vi "test_Add Response_Variable Names Error.vi"(8 "error in (no error)":errorcluster, 11 "TestCase in":refnum<class "Instrument Addon Scripting API Messages Unit Tests.lvclass">) -> (0 "error out":errorcluster, 3 "TestCase out":refnum<class "Instrument Addon Scripting API Messages Unit Tests.lvclass">)   [LabVIEW 2018, in "Instrument Addon Scripting API Messages Unit Tests.lvclass"]
uses:
  Instrument Addon Scripting API Messages Unit Tests.lvclass
  APIs/Scripting API/TypeDefs/Wait Response Settings.ctl
  APIs/Scripting API/TypeDefs/Linked Channel.ctl
  <vilib>/NI Veristand/Custom Device API/Custom Device Item Ref.ctl
  Addon/Addon Shared/SubVIs/Constants.vi
  <vilib>/NI/NI VeriStand Advanced SysDef API/_SubVIs/SysDef.Search.GUID.vi
  APIs/Scripting API/Messages/Add Response - Wait (sec).vi
  <vilib>/addons/_JKI Toolkits/VI Tester/TestCase.llb/TestCase.lvclass
  Instrument Addon Scripting API Test Assets/Instrument Addon Scripting API Test Assets.lvclass
  APIs/Scripting API/Instrument Addon Scripting API.lvlib
  <vilib>/NI Veristand/Custom Device API/Custom Device API.lvlib
  <vilib>/NI/NI VeriStand Advanced SysDef API/SysDef API/Advanced System Definition.lvlib
  Addon/Addon Shared/Instrument Addon Shared.lvlib
  C:/Program Files (x86)/National Instruments/LabVIEW 2018/vi.lib/addons/_JKI Toolkits/VI Tester/TestCase.llb/TestCase.lvclass
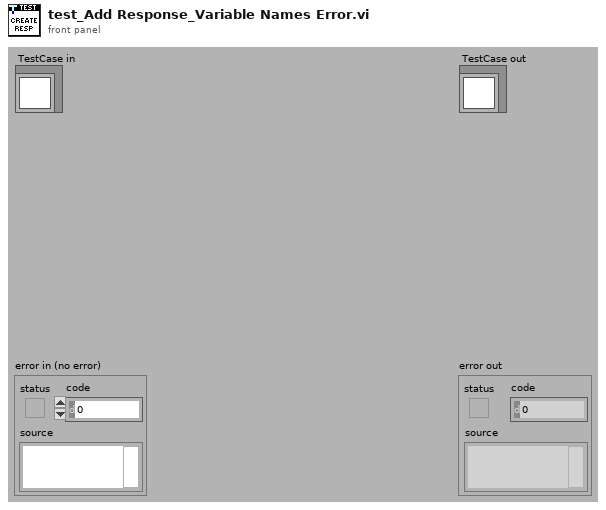
[diagram p1: front panel]
types:
  T1 = typedef "Instrument Addon Scripting API.lvlib/Wait Response Settings.ctl" = cluster{"Response Format":string, "Linked Channels":T2[], "Wait value (sec)":dbl, "Use Wait Channel":bool, "Channel Refnum":T3}
  T2 = typedef "Instrument Addon Scripting API.lvlib/Linked Channel.ctl" = cluster{"Variable Name":string, "Channel Refnum":T3}
  T3 = typedef "Custom Device API.lvlib/Custom Device Item Ref.ctl" = u64
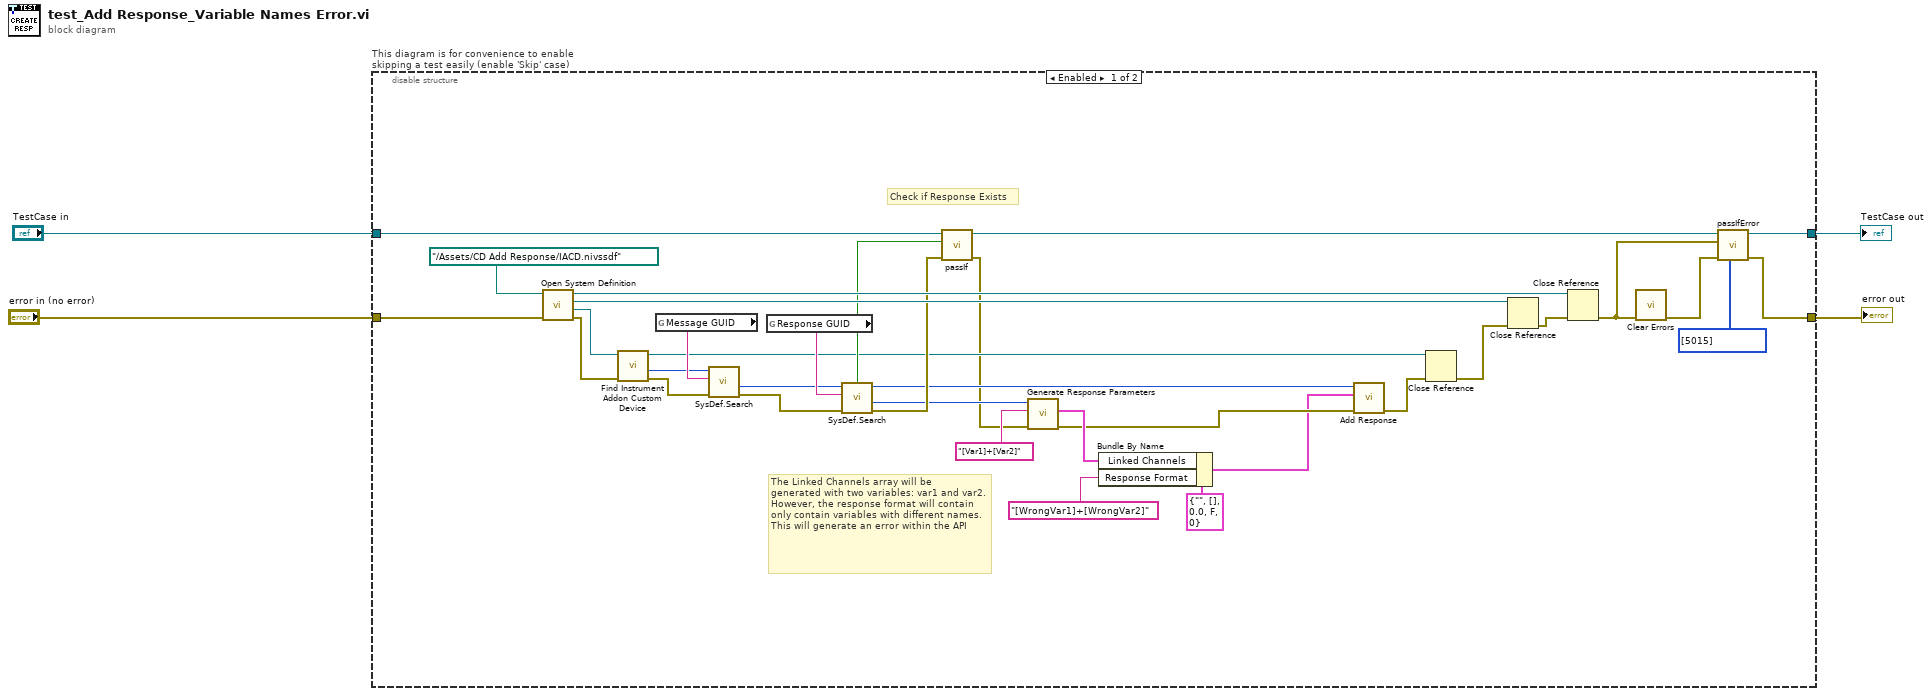
[diagram p0: block diagram]
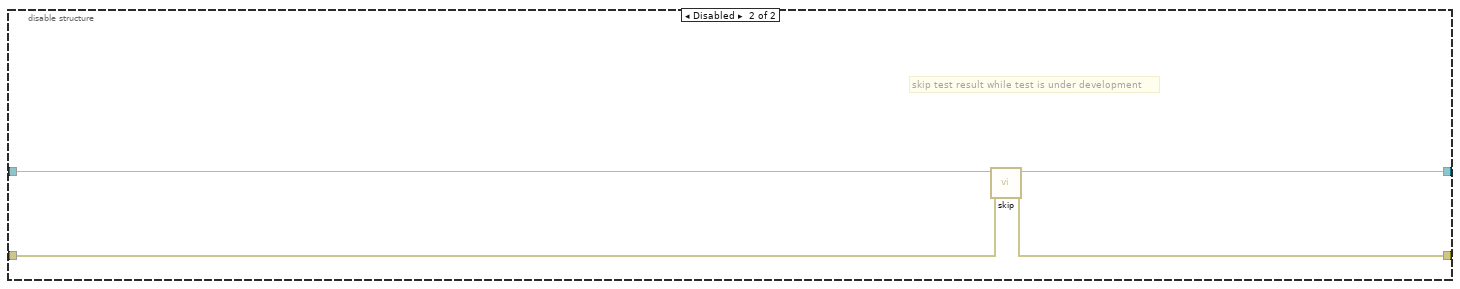
[diagram p2: hidden frame]
diagram:
  n1 = disable-structure "This diagram is for convenience to enable skipping a test easily (enable 'Skip' case)" shown="Enabled" {
    disable-tunnel: "TestCase in" -> [w29 w42]
    disable-tunnel: [w24 w40] -> w1
    disable-tunnel: [w23 w41] -> w3
    disable-tunnel: "error in (no error)" -> [w37 w39]
    frame Enabled {
      # "The Linked Channels array will be \ngenerated with two variables: var1 and var2. However, the response format will contain only contain variables with different names. This will generate an error within the API"
      # "Check if Response Exists"
      n2 = call "Open System Definition.vi"("error in (no error)"=w37, "System Definition File"=path "../Assets/CD Add Response/IACD.nivssdf" ("SDF file")) -> ("error out"=w35:errorcluster, "Target Refnum"=w34:refnum<k24>, "Root Refnum"=w33:refnum<k24>, "System Definition Refnum"=w32:refnum<k24>)  [unwired: 6 in]
      n3 = call "Find Instrument Addon Custom Device.vi"("error in"=w35, "target in"=w34) -> ("error out"=w18:errorcluster, "NodeID"=w17:u64, "target out"=w13:refnum<k24>)  [unwired: 7 in]
      n4 = global read "Constants.vi" "Message GUID"() -> (w19:string)
      n5 = call-poly <vilib>:"SysDef.Search.vi"("error in (no error)"=w18, "GUID"=w19, "nodeID"=w17) -> ("error out"=w15:errorcluster, "Value out"=w16:u64)  [unwired: 5 in, 2 out]
      n6 = global read "Constants.vi" "Response GUID"() -> (w30:string)
      n7 = call-poly <vilib>:"SysDef.Search.vi"("error in (no error)"=w15, "GUID"=w30, "nodeID"=w16) -> ("error out"=w14:errorcluster, "Value out"=w11:u64, "nodeID out"=w12:u64, "Found?"=w28:bool)  [unwired: 5 in]
      n8 = call-dynamic "passIf.vi"("error in (no error)"=w14, "pass"=w28, "TestCase in"=w29) -> ("error out"=w9:errorcluster, "TestCase out"=w25:refnum<class "Instrument Addon Scripting API Messages Unit Tests.lvclass">)  [unwired: 7 in]
      n9 = call "Generate Response Parameters.vi"("Error In"=w9, "Response String"="[Var1]+[Var2]" ("Response Format"), "Response Channel in"=w11) -> ("Error Out"=w6:errorcluster, "Linked Channels"=w8:T2[])  [unwired: 5 in, 2 out]
      n10 = Bundle By Name(cluster=T1 {"Response Format"="", "Linked Channels"=[], "Wait value (sec)"=0.0, "Use Wait Channel"=FALSE, "Channel Refnum"=0} ("Settings"), "Linked Channels"=w8, "Response Format"="[WrongVar1]+[WrongVar2]") -> (w5:T1)
      n11 = call-poly "Add Response.vi"("error in (no error)"=w6, "Settings"=w5, "Message in"=w12) -> ("error out"=w26:errorcluster)  [unwired: 7 in, 1 out]
      n12 = Close Reference(reference=w13, error in (no error)=w26) -> (error out=w36:errorcluster)
      n13 = Close Reference(reference=w33, error in (no error)=w36) -> (error out=w31:errorcluster)
      n14 = Close Reference(reference=w32, error in (no error)=w31) -> (error out=w21:errorcluster)
      n15 = call <vilib>:"Clear Errors.vi"("error in (no error)"=w21) -> ("error out"=w20:errorcluster)  [unwired: 5 in, 1 out]
      n16 = call-dynamic "passIfError.vi"("passing error codes (default = any error code)"=i32[] [5015], "error in (no error)"=w20, "error"=w21, "TestCase in"=w25) -> ("error out"=w23:errorcluster, "TestCase out"=w24:refnum<class "Instrument Addon Scripting API Messages Unit Tests.lvclass">)  [unwired: 6 in]
    }
    frame Disabled {
      # "skip test result while test is under development"
      n17 = call <vilib>:"skip.vi"("error in (no error)"=w39, "TestCase in"=w42) -> ("error out"=w41:errorcluster, "TestCase out"=w40:refnum<class "Instrument Addon Scripting API Messages Unit Tests.lvclass">)  [unwired: 8 in]
    }
  }
  "error out" <- w3
  "TestCase out" <- w1
